vi "FTPSync_Configure.vi"(8 "error in (no error)":errorcluster, 10 "?":T1={"address"="127.0.0.1", "remote port"=21, "userName"="user", "passWord"="password", "RootDir"="/"}, 11 "FTPProtocol in":refnum<class "FTPProtocol.lvclass">) -> (0 "error out":errorcluster, 3 "FTPProtocol out":refnum<class "FTPProtocol.lvclass">)   [LabVIEW 2020, in "CSM-FileSync.lvlib" / "FTPProtocol.lvclass"]
uses:
  FTPProtocol.lvclass
  FTPProtocol.lvclass/FTPProtocol.ctl
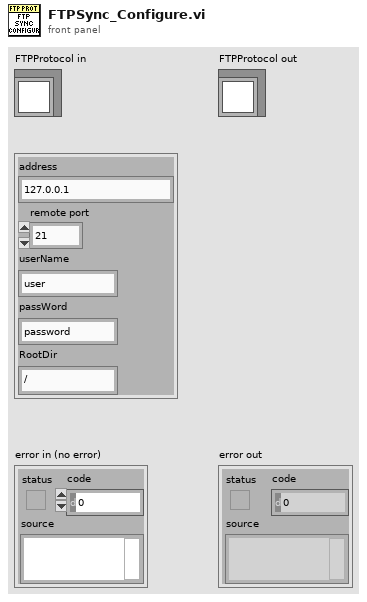
[diagram p1: front panel]
types:
  T1 = cluster{"address":string, "remote port":u16, "userName":string, "passWord":string, "RootDir":string}
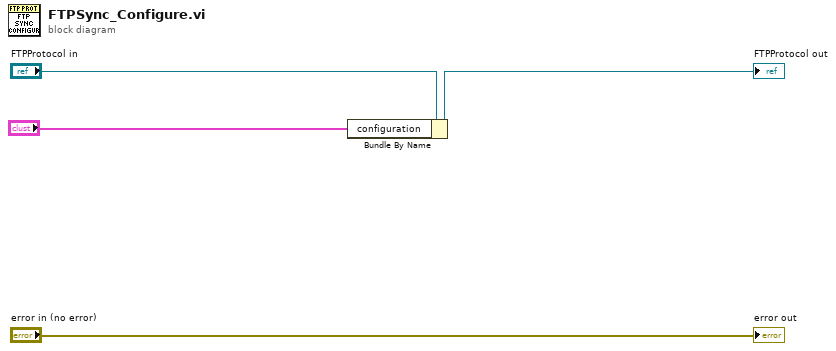
[diagram p0: block diagram]
diagram:
  n1 = Bundle By Name(cluster="FTPProtocol in", "configuration"="?") -> (→"FTPProtocol out":refnum<class "FTPProtocol.lvclass">)
  "error out" <- "error in (no error)"
